vi "PH_IEEE1394Camera.set Numeric Cam Attribute Tip Strip.vi"(1 "Minimum":u32, 2 "Maximum":u32, 3 "Attribute":string) -> (0 "Tip Strip":string)   [LabVIEW 2014, in "PH_IEEE1394Camera.lvlib"]
doc: "This VI sets a numeric Cam Attribute tip strip."
uses:
  PH_IEEE1394Camera.lvlib
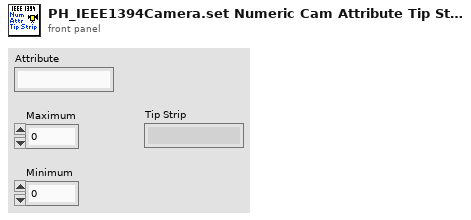
[diagram p1: front panel]
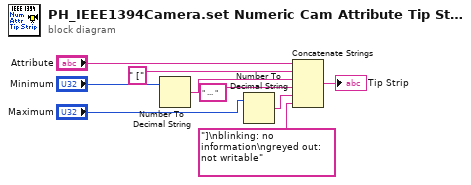
[diagram p0: block diagram]
diagram:
  n1 = Number To Decimal String(number="Minimum") -> (decimal integer string=w5:string)  [unwired: 1 in]
  n2 = Number To Decimal String(number="Maximum") -> (decimal integer string=w6:string)  [unwired: 1 in]
  n3 = Concatenate Strings("Attribute", " [" ("string"), w5, " ... " ("string"), w6, "]\nblinking: no information\ngreyed out: not writable") -> (→"Tip Strip":string)
